vi "Fdx Statistics Table.vi"(11 "GlobalStat Out":T1) -> (3 "Table Control":string[][](table))   [LabVIEW 2020, in "AIM664LV.lvlib"]
doc: "Converts a GlobalStat cluster into a table."
uses:
  AIM664LV.lvlib
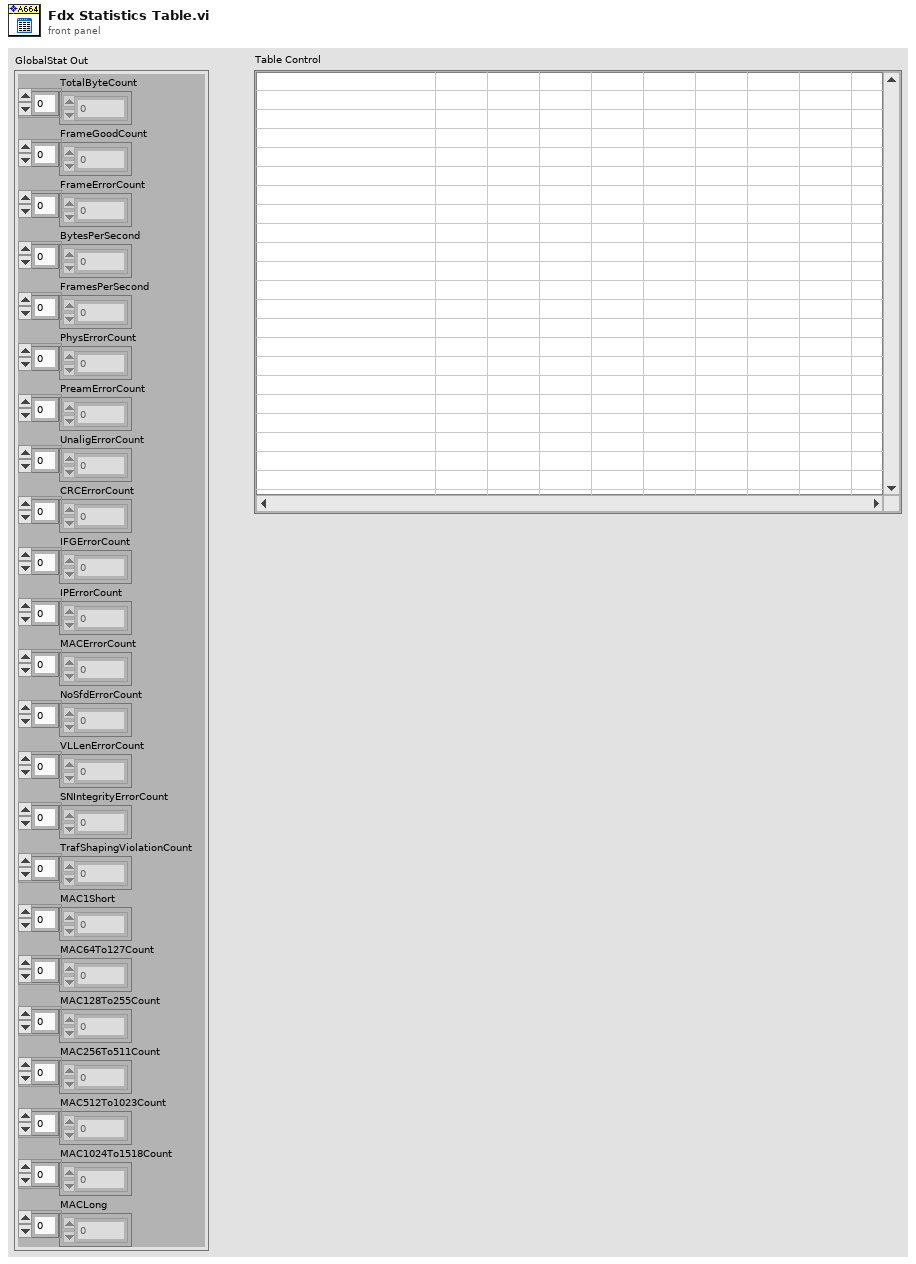
[diagram p1: front panel]
types:
  T1 = cluster{"TotalByteCount":u32[], "FrameGoodCount":u32[], "FrameErrorCount":u32[], "BytesPerSecond":u32[], "FramesPerSecond":u32[], "PhysErrorCount":u32[], "PreamErrorCount":u32[], "UnaligErrorCount":u32[], "CRCErrorCount":u32[], "IFGErrorCount":u32[], "IPErrorCount":u32[], "MACErrorCount":u32[], "NoSfdErrorCount":u32[], "VLLenErrorCount":u32[], "SNIntegrityErrorCount":u32[], "TrafShapingViolationCount":u32[], "MAC1Short":u32[], "MAC64To127Count":u32[], "MAC128To255Count":u32[], "MAC256To511Count":u32[], "MAC512To1023Count":u32[], "MAC1024To1518Count":u32[], "MACLong":u32[]}
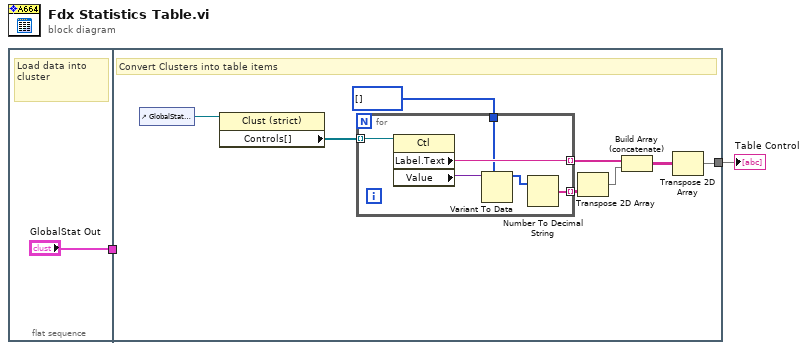
[diagram p0: block diagram]
diagram:
  n1 = flat-sequence {
    tunnel: ["GlobalStat Out"] -> w1
    tunnel: [w4] -> w2
    tunnel: w1 -> [_]
    frame #0 {
      # "Load data into cluster"
    }
    frame #1 {
      # "Convert Clusters into table items"
      n2 = control-ref of="GlobalStat Out"() -> (w10:refnum<vi>)
      n3 = property on="Property Node" class="Clust (strict)"(reference=w10) -> ("Controls[]"=w11:refnum<vi>[])  [unwired: 1 in, 2 out]
      n4 = for {
        tunnel: w11 -> [w17] mode=indexing
        tunnel: [w16] -> w8 mode=indexing
        tunnel: u32[] [] ("TotalByteCount") -> [w14]
        tunnel: [w12] -> w7 mode=indexing
        n5 = property class="Ctl"(reference=w17) -> ("Label.Text"=w16:string, "Value"=w15:variant)  [unwired: 1 in, 2 out]
        n6 = Variant To Data(type=w14, Variant=w15) -> (data=w13:u32[])  [unwired: 1 in, 1 out]
        n7 = Number To Decimal String(number=w13) -> (decimal integer string=w12:string[])  [unwired: 1 in]
      }
      n8 = Transpose 2D Array(2D array=w7) -> (transposed array=w5:string[][])
      n9 = Build Array (concatenate)(w8, w5) -> (w6:string[][])
      n10 = Transpose 2D Array(2D array=w6) -> (transposed array=w4:string[][])
    }
  }
  "Table Control" <- w2
